vi "Filter Wheel Arduino Calc Distance.vi"(8 "error in (no error)":errorcluster, 10 "To Position":i32, 11 "From Pos":i32) -> (0 "error out":errorcluster, 2 "Direction":string, 3 "Counts":u32)   [LabVIEW 2021]
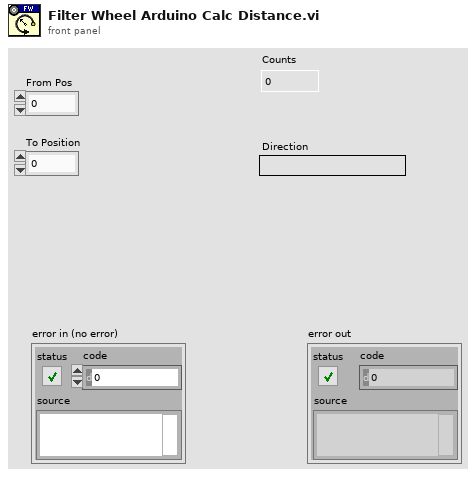
[diagram p1: front panel]
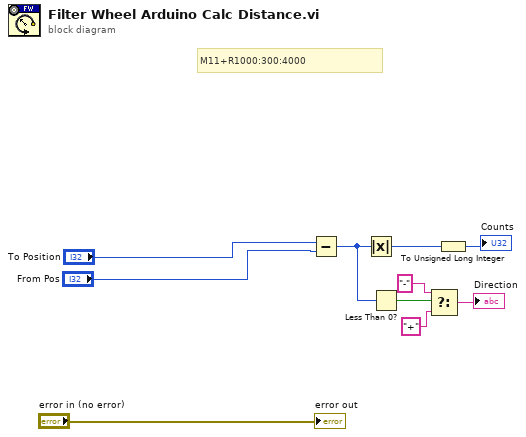
[diagram p0: block diagram]
diagram:
  # "M11+R1000:300:4000"
  n1 = Subtract(x="To Position", y="From Pos") -> (x-y=w7:i32)
  n2 = Absolute Value(x=w7) -> (abs(x)=w8:i32)
  n3 = Less Than 0?(x=w7) -> (x < 0?=w6:bool)
  n4 = Select(t="-", s=w6, f="+") -> (s? t:f=→"Direction":string)
  n5 = To Unsigned Long Integer(number=w8) -> (unsigned 32bit integer=→"Counts":u32)
  "error out" <- "error in (no error)"
